vi "JSON Editor.vi"() -> ()   [LabVIEW 2017]
uses:
  Advanced LabVIEW Variant APIs/Advanced Variant Tools.lvlib
panel:
  in  "load":bool
  in  "error in (no error)":errorcluster
  in  "stop":bool
  in  "pretty print":bool
  in  "JSON String":string
  in  "Tree":string(tree)
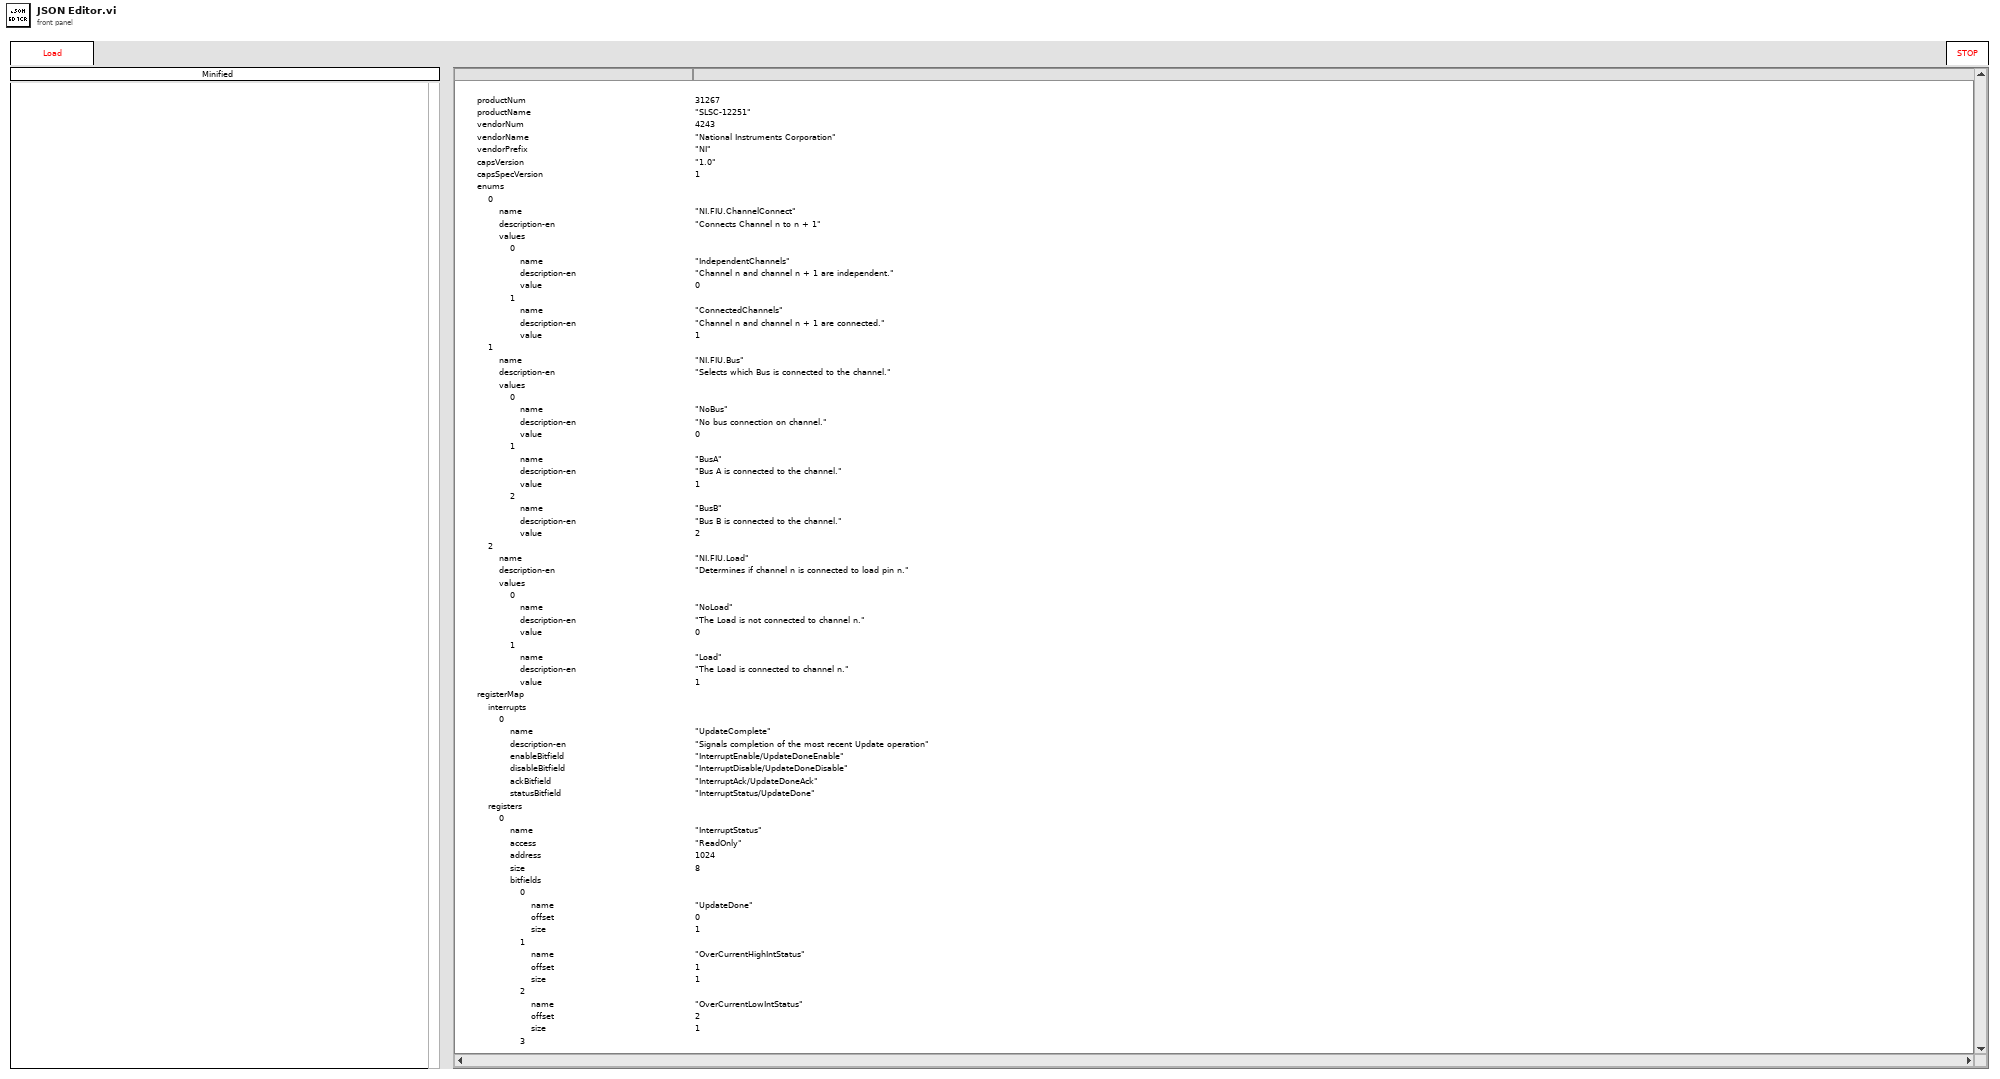
[diagram p1: front panel]
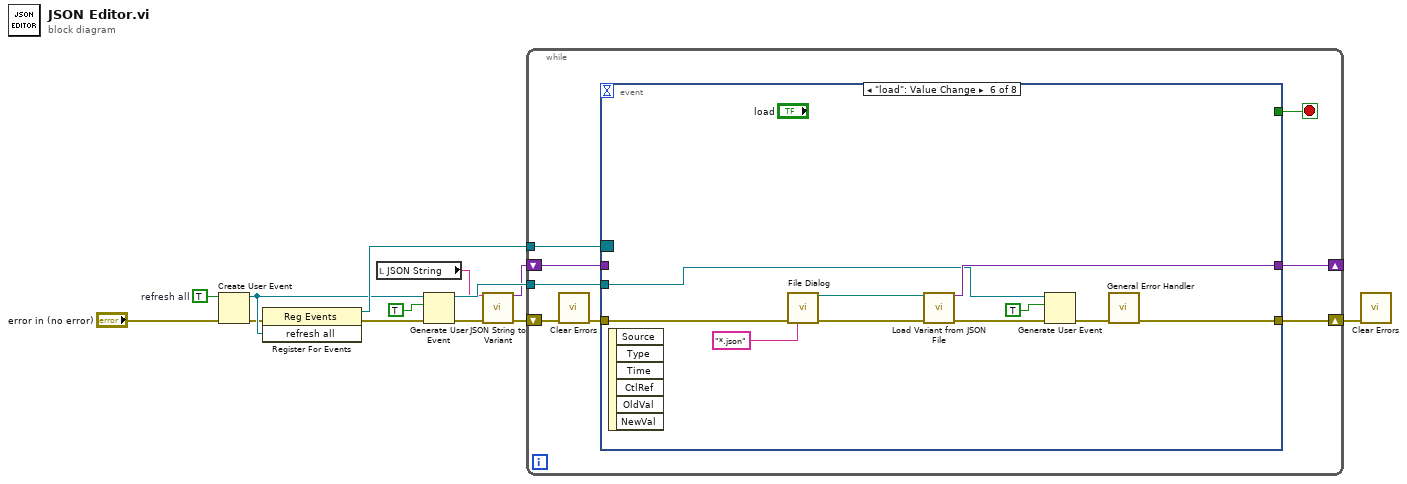
[diagram p0: block diagram]
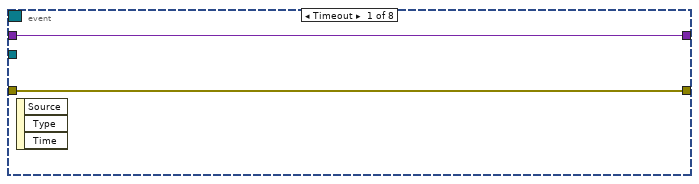
[diagram p2: hidden frame]
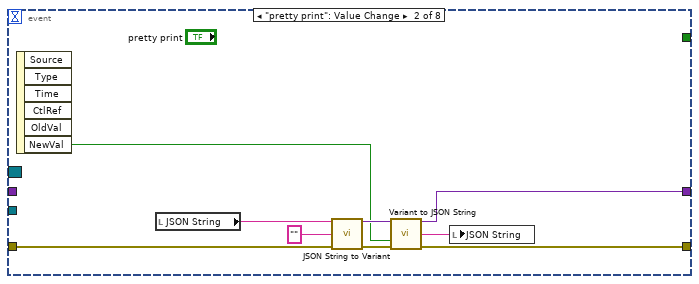
[diagram p3: hidden frame]
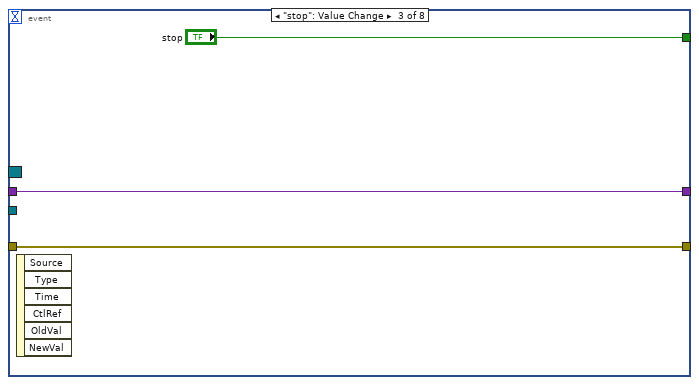
[diagram p4: hidden frame]
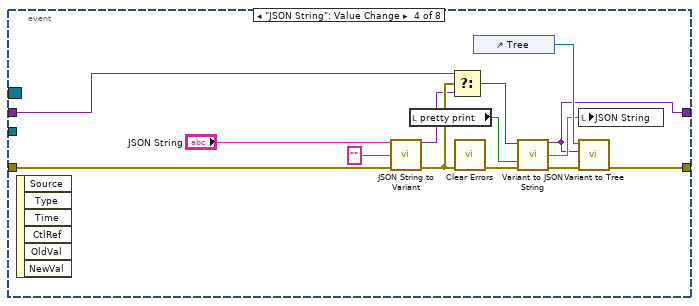
[diagram p5: hidden frame]
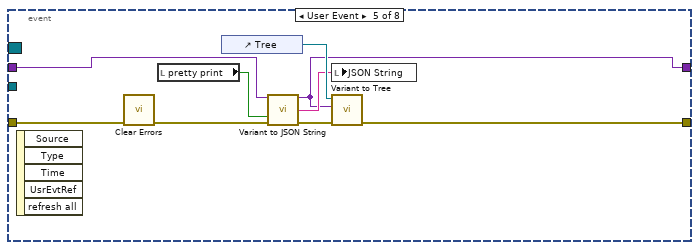
[diagram p6: hidden frame]
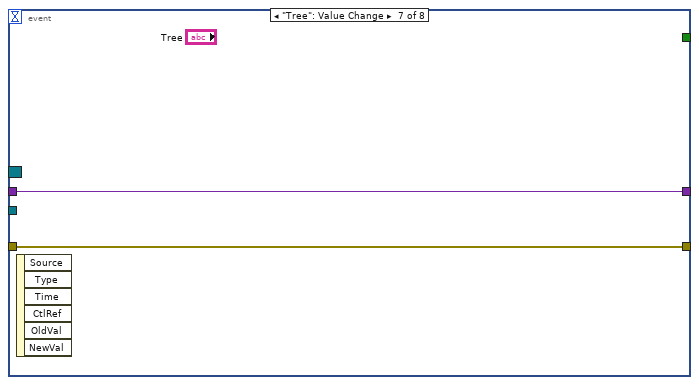
[diagram p7: hidden frame]
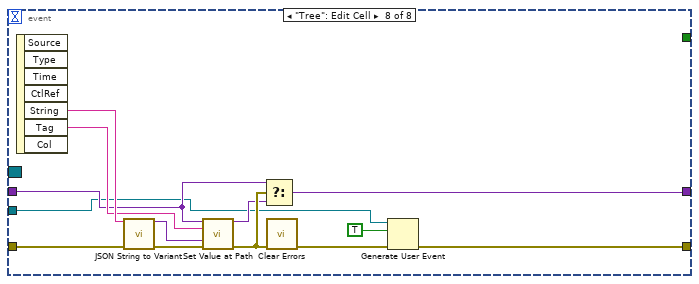
[diagram p8: hidden frame]
diagram:
  w12 = TRUE  # refresh all
  n1 = Create User Event(user event datatype=w12, error in="error in (no error)") -> (user event=w10:refnum<user-event>, error out=w7:errorcluster)
  n2 = register-events(error in=w7, w10) -> (reference out=w11:refnum<event-registration>, error out=w6:errorcluster)  [unwired: 1 in]
  n3 = local read "JSON String"() -> (w4:string)
  n4 = Generate User Event(user event=w10, event data cluster=TRUE ("event data"), error in=w6) -> (user event out=w5:refnum<user-event>, error out=w2:errorcluster)  [unwired: 1 in]
  n5 = call "JSON String to Variant.vi"("JSON String"=w4, "error in (no error)"=w2) -> ("Variant out"=w3:variant, "error out"=w1:errorcluster)  [unwired: 12 in]
  n6 = while {
    shift-right: [w19] -> w13
    shift-left: w1 -> [w20]
    shift-right: [w17] -> _
    shift-left: w3 -> [w16]
    tunnel: w11 -> [w15]
    tunnel: w5 -> [w14]
    stop <- w21 stop-if-true
    n7 = call <vilib>:"Clear Errors.vi"("error in (no error)"=w20) -> ("error out"=w18:errorcluster)  [unwired: 5 in, 1 out]
    n8 = event shown="[5] \"load\": Value Change" {
      selector: w15 -> [_ _ _ _ _ _ _ _]
      dyn-events: _ -> [_ _ _ _ _ _ _ _]
      timeout: _ -> [_ _ _ _ _ _ _ _]
      tunnel: [_ _ "stop" _ _ _ _ _] -> w21
      tunnel: w18 -> [w23 w26 w34 w45 w56 w65 w70 w81]
      tunnel: [w23 w25 w34 w47 w58 w63 w70 w71] -> w19
      tunnel: w16 -> [w22 _ w33 w39 w51 _ w69 w77]
      tunnel: [w22 w24 w33 w41 w52 w68 w69 w75] -> w17
      tunnel: w14 -> [_ _ _ _ _ w60 _ w73]
      event Timeout {
        n9 = event-data() -> ()  [unwired: 1 in, 3 out]
      }
      event "pretty print": Value Change {
        n10 = event-data() -> ("NewVal"=w29:bool)  [unwired: 1 in, 5 out]
        n11 = local read "JSON String"() -> (w31:string)
        n12 = call "JSON String to Variant.vi"("JSON String"=w31, "Top-Level Control Name"="", "error in (no error)"=w26) -> ("Variant out"=w30:variant, "error out"=w28:errorcluster)  [unwired: 11 in]
        n13 = call "Variant to JSON String.vi"("Variant in"=w30, "pretty print? (F)"=w29, "error in (no error)"=w28) -> ("Variant out"=w24:variant, "String"=w27:string, "error out"=w25:errorcluster)  [unwired: 10 in]
        n14 = local write "JSON String"(w27) -> ()
      }
      event "stop": Value Change {
        n15 = event-data() -> ()  [unwired: 1 in, 6 out]
      }
      event "JSON String": Value Change {
        n16 = event-data() -> ()  [unwired: 1 in, 6 out]
        n17 = call "JSON String to Variant.vi"("JSON String"="JSON String", "Top-Level Control Name"="", "error in (no error)"=w45) -> ("Variant out"=w38:variant, "error out"=w40:errorcluster)  [unwired: 11 in]
        n18 = local read "pretty print"() -> (w44:bool)
        n19 = Select(t=w39, s=w40, f=w38) -> (s? t:f=w37:variant)
        n20 = call <vilib>:"Clear Errors.vi"("error in (no error)"=w40) -> ("error out"=w36:errorcluster)  [unwired: 5 in, 1 out]
        n21 = control-ref of="Tree"() -> (w46:refnum<vi>)
        n22 = call "Variant to JSON String.vi"("Variant in"=w37, "pretty print? (F)"=w44, "error in (no error)"=w36) -> ("Variant out"=w41:variant, "String"=w43:string, "error out"=w42:errorcluster)  [unwired: 10 in]
        n23 = local write "JSON String"(w43) -> ()
        n24 = call "Variant to Tree.vi"("error in (no error)"=w42, "Variant"=w41, "TreeControl in"=w46) -> ("error out"=w47:errorcluster)  [unwired: 8 in]
      }
      event User Event {
        n25 = event-data() -> ()  [unwired: 1 in, 5 out]
        n26 = call <vilib>:"Clear Errors.vi"("error in (no error)"=w56) -> ("error out"=w50:errorcluster)  [unwired: 5 in, 1 out]
        n27 = local read "pretty print"() -> (w55:bool)
        n28 = control-ref of="Tree"() -> (w57:refnum<vi>)
        n29 = call "Variant to JSON String.vi"("Variant in"=w51, "pretty print? (F)"=w55, "error in (no error)"=w50) -> ("Variant out"=w52:variant, "String"=w54:string, "error out"=w53:errorcluster)  [unwired: 10 in]
        n30 = local write "JSON String"(w54) -> ()
        n31 = call "Variant to Tree.vi"("error in (no error)"=w53, "Variant"=w52, "TreeControl in"=w57) -> ("error out"=w58:errorcluster)  [unwired: 8 in]
      }
      event "load": Value Change {
        n32 = event-data() -> ()  [unwired: 1 in, 6 out]
        n33 = call "File Dialog"("error in"=w65, "pattern (all files)"="*.json" ("pattern label")) -> ("selected path"=w67:path, "error out"=w64:errorcluster)  [unwired: 10 in, 2 out]
        n34 = call "Load Variant from JSON File.vi"("file path"=w67, "error in"=w64) -> ("Variant out"=w68:variant, "error out"=w62:errorcluster)  [unwired: 12 in]
        n35 = Generate User Event(user event=w60, event data cluster=TRUE ("event data"), error in=w62) -> (error out=w61:errorcluster)  [unwired: 1 in, 1 out]
        n36 = call <vilib>:"General Error Handler.vi"("error in (no error)"=w61) -> ("error out"=w63:errorcluster)  [unwired: 10 in, 4 out]
      }
      event "Tree": Value Change {
        n37 = event-data() -> ()  [unwired: 1 in, 6 out]
      }
      event "Tree": Edit Cell {
        n38 = event-data() -> ("String"=w83:string, "Tag"=w79:string)  [unwired: 1 in, 5 out]
        n39 = call "JSON String to Variant.vi"("JSON String"=w83, "error in (no error)"=w81) -> ("Variant out"=w80:variant, "error out"=w82:errorcluster)  [unwired: 12 in]
        n40 = call "Set Value at Path.vi"("Variant in"=w77, "Path String"=w79, "Element in"=w80, "error in (no error)"=w82) -> ("Variant out"=w76:variant, "error out"=w78:errorcluster)  [unwired: 10 in]
        n41 = Select(t=w77, s=w78, f=w76) -> (s? t:f=w75:variant)
        n42 = call <vilib>:"Clear Errors.vi"("error in (no error)"=w78) -> ("error out"=w74:errorcluster)  [unwired: 5 in, 1 out]
        n43 = Generate User Event(user event=w73, event data cluster=TRUE ("event data"), error in=w74) -> (error out=w71:errorcluster)  [unwired: 1 in, 1 out]
      }
    }
  }
  n44 = call <vilib>:"Clear Errors.vi"("error in (no error)"=w13) -> ()  [unwired: 5 in, 2 out]
